vi "AlliGator MCP Voltage to Gain.vi"(9 "MCP Parameters":T1={"G0"=3.0, "A"=4.052e-06, "V0"=174.3, "B"=0.0422, "g"=0.322}, 11 "MCP Voltage":dbl) -> (3 "Gain":dbl)   [LabVIEW 2021, in "AlliGator Intensity Corrections.lvlib"]
doc: "Heuristic fit of the relationship between effective ICCD gain G and MCP voltage V_MCP.\n\nThe function used is a stretched exponential with vertical and horizontal offsets.\n\nParameters need to be fitted independetly with a G(V_MCP) series."
uses:
  AlliGator Intensity Corrections.lvlib
  AlliGator MCP Parameters.ctl
panel:
  # "see the AlliGator License on the block diagram (Ctrl+E or Window:Show Block Diagram)"
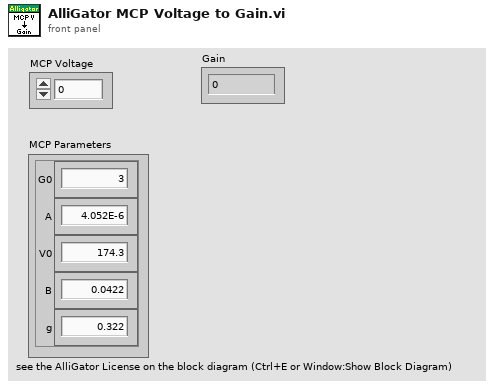
[diagram p1: front panel]
types:
  T1 = typedef "AlliGator Intensity Corrections.lvlib/AlliGator MCP Parameters.ctl" = cluster{"G0":dbl, "A":dbl, "V0":dbl, "B":dbl, "g":dbl}
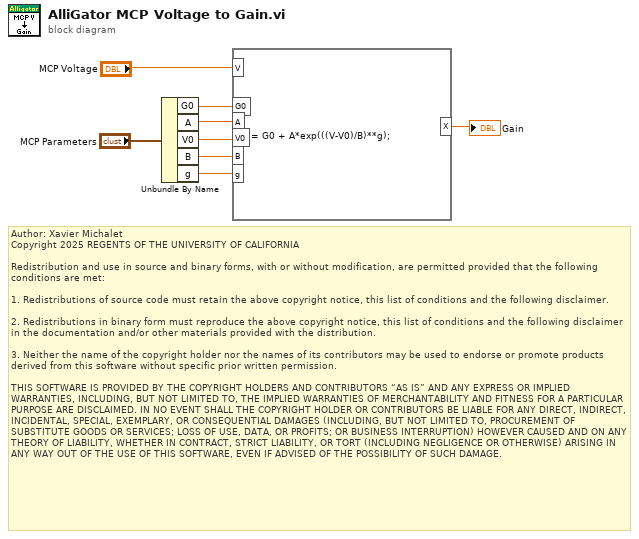
[diagram p0: block diagram]
diagram:
  # "Author: Xavier Michalet\nCopyright 2025 REGENTS OF THE UNIVERSITY OF CALIFORNIA\n\nRedistribution and use in source and binary forms, with or without modification, are permitted provided that the following conditions are met:\n\n1. Redistributions of source code must retain the above copyright notice, this list of conditions and the following disclaimer.\n\n2. Redistributions in binary form must reproduce the above copyright notice, this list of conditions and the following disclaimer in the documentation and/or other materials provided with the distribution.\n\n3. Neither the name of the copyright holder nor the names of its contributors may be used to endorse or promote products derived from this software without specific prior written permission.\n\nTHIS SOFTWARE IS PROVIDED BY THE COPYRIGHT HOLDERS AND CONTRIBUTORS “AS IS” AND ANY EXPRESS OR IMPLIED WARRANTIES, INCLUDING, BUT NOT LIMITED TO, THE IMPLIED WARRANTIES OF MERCHANTABILITY AND FITNESS FOR A PARTICULAR PURPOSE ARE DISCLAIMED. IN NO EVENT SHALL THE COPYRIGHT HOLDER OR CONTRIBUTORS BE LIABLE FOR ANY DIRECT, INDIRECT, INCIDENTAL, SPECIAL, EXEMPLARY, OR CONSEQUENTIAL DAMAGES (INCLUDING, BUT NOT LIMITED TO, PROCUREMENT OF SUBSTITUTE GOODS OR SERVICES; LOSS OF USE, DATA, OR PROFITS; OR BUSINESS INTERRUPTION) HOWEVER CAUSED AND ON ANY THEORY OF LIABILITY, WHETHER IN CONTRACT, STRICT LIABILITY, OR TORT (INCLUDING NEGLIGENCE OR OTHERWISE) ARISING IN ANY WAY OUT OF THE USE OF THIS SOFTWARE, EVEN IF ADVISED OF THE POSSIBILITY OF SUCH DAMAGE."
  n1 = Unbundle By Name("MCP Parameters") -> ("G0"=w5:dbl, "A"=w4:dbl, "V0"=w3:dbl, "B"=w2:dbl, "g"=w1:dbl)
  n2 = formula code="X = G0 + A*exp(((V-V0)/B)**g);"("V"="MCP Voltage", "G0"=w5, "A"=w4, "V0"=w3, "B"=w2, "g"=w1) -> ("X"=→"Gain":dbl)
